vi "activate lib.vi"() -> ()   [LabVIEW 2009, in "pc control room shared var.lvlib"]
uses:
  pc control room shared var.lvlib
panel:
  out "Boolean":bool
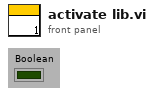
[diagram p1: front panel]
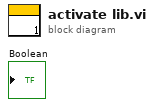
[diagram p0: block diagram]
diagram:
